vi "NewGameBoard.vi"(1 "Grid Size":T1, 2 "Color Box":u32(colorbox), 5 "error in (no error)":errorcluster) -> (14 "object out":refnum<class "Game Board.lvclass">, 19 "error out":errorcluster)   [LabVIEW 2021, in "Game Board.lvclass"]
uses:
  Game Board.lvclass
  Coordinates.ctl
  Game Board.lvclass/Game Board.ctl
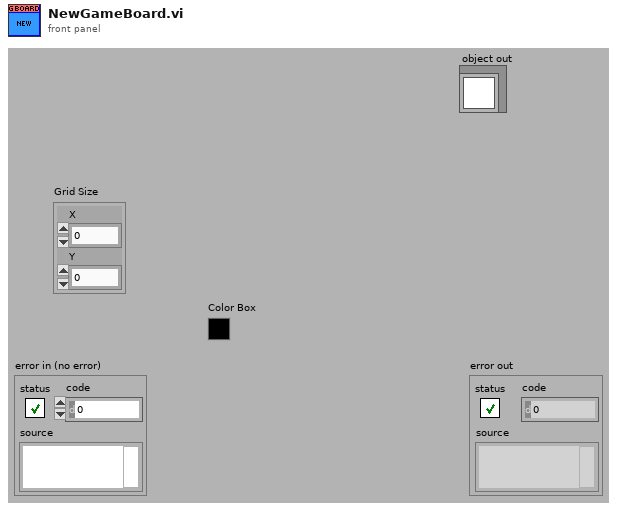
[diagram p1: front panel]
types:
  T1 = typedef "Coordinates.ctl" = cluster{"X":i32, "Y":i32}
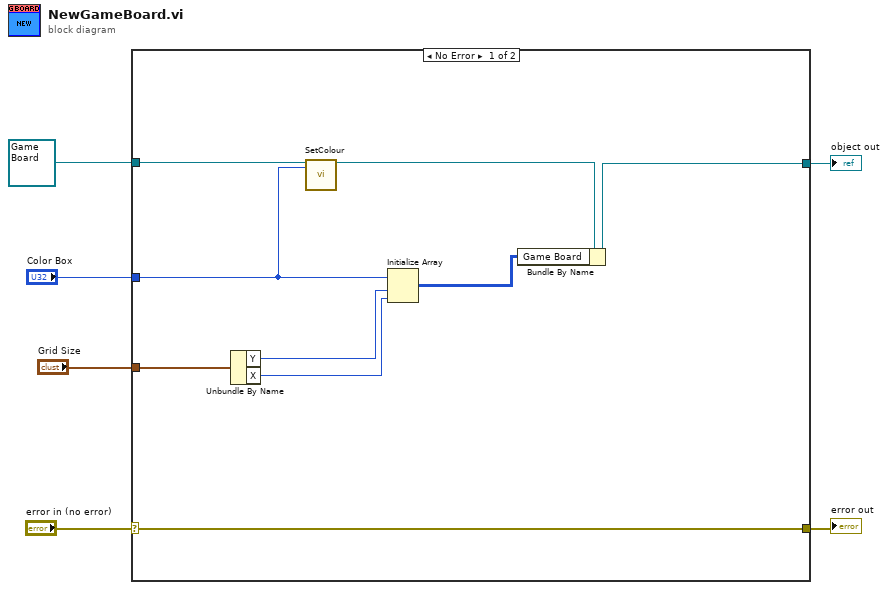
[diagram p0: block diagram]
diagram:
  n1 = case shown="No Error" "error in (no error)" {
    selector: "error in (no error)" -> [w15 w17]
    tunnel: [w15 w17] -> w5
    tunnel: [w14 w16] -> w4
    tunnel: refnum<class "Game Board.lvclass"> refnum ("Game Board") -> [w13 w16]
    tunnel: "Color Box" -> [w8 _]
    tunnel: "Grid Size" -> [w11 _]
    frame No Error {
      n2 = Unbundle By Name(w11) -> ("Y"=w10:i32, "X"=w9:i32)
      n3 = call-dynamic "SetColour.vi"("object in"=w13, "Colour"=w8) -> ("object out"=w12:refnum<class "Game Board.lvclass">)  [unwired: 16 in, 1 out]
      n4 = Initialize Array(w8, w10, w9) -> (w7:u32[][])
      n5 = Bundle By Name(cluster=w12, "Game Board"=w7) -> (w14:refnum<class "Game Board.lvclass">)
    }
    frame Error {
    }
  }
  "error out" <- w5
  "object out" <- w4
